vi "lv channel free.vi"(8 "error in (no error)":errorcluster, 11 "channel handle":i32) -> (0 "error out":errorcluster)   [LabVIEW 2026]
uses:
  bin/nominalClient_64.dll
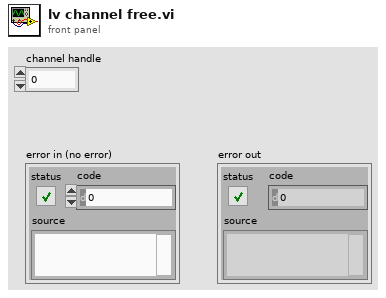
[diagram p1: front panel]
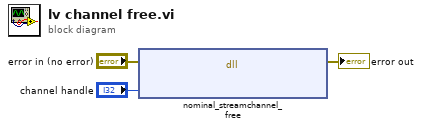
[diagram p0: block diagram]
diagram:
  n1 = dll-call lib="C:/sw/nominal-c/bin/nominalClient_64.dll" fn="nominal_streamchannel_free"(error in="error in (no error)", "channel handle"="channel handle") -> (error out=→"error out":errorcluster)  [unwired: 4 in, 1 out]
